vi "GetClampMAXResultValue.vi"(8 "error in (no error)":errorcluster, 9 "data":T1, 11 "Analysis_Clamp MAX_Parameter":T2) -> (0 "error out":errorcluster, 3 "ResultValues":string[](array[string]))   [LabVIEW 2019]
uses:
  Controls/Clamp MAX/Analysis_Clamp MAX_Parameter.ctl
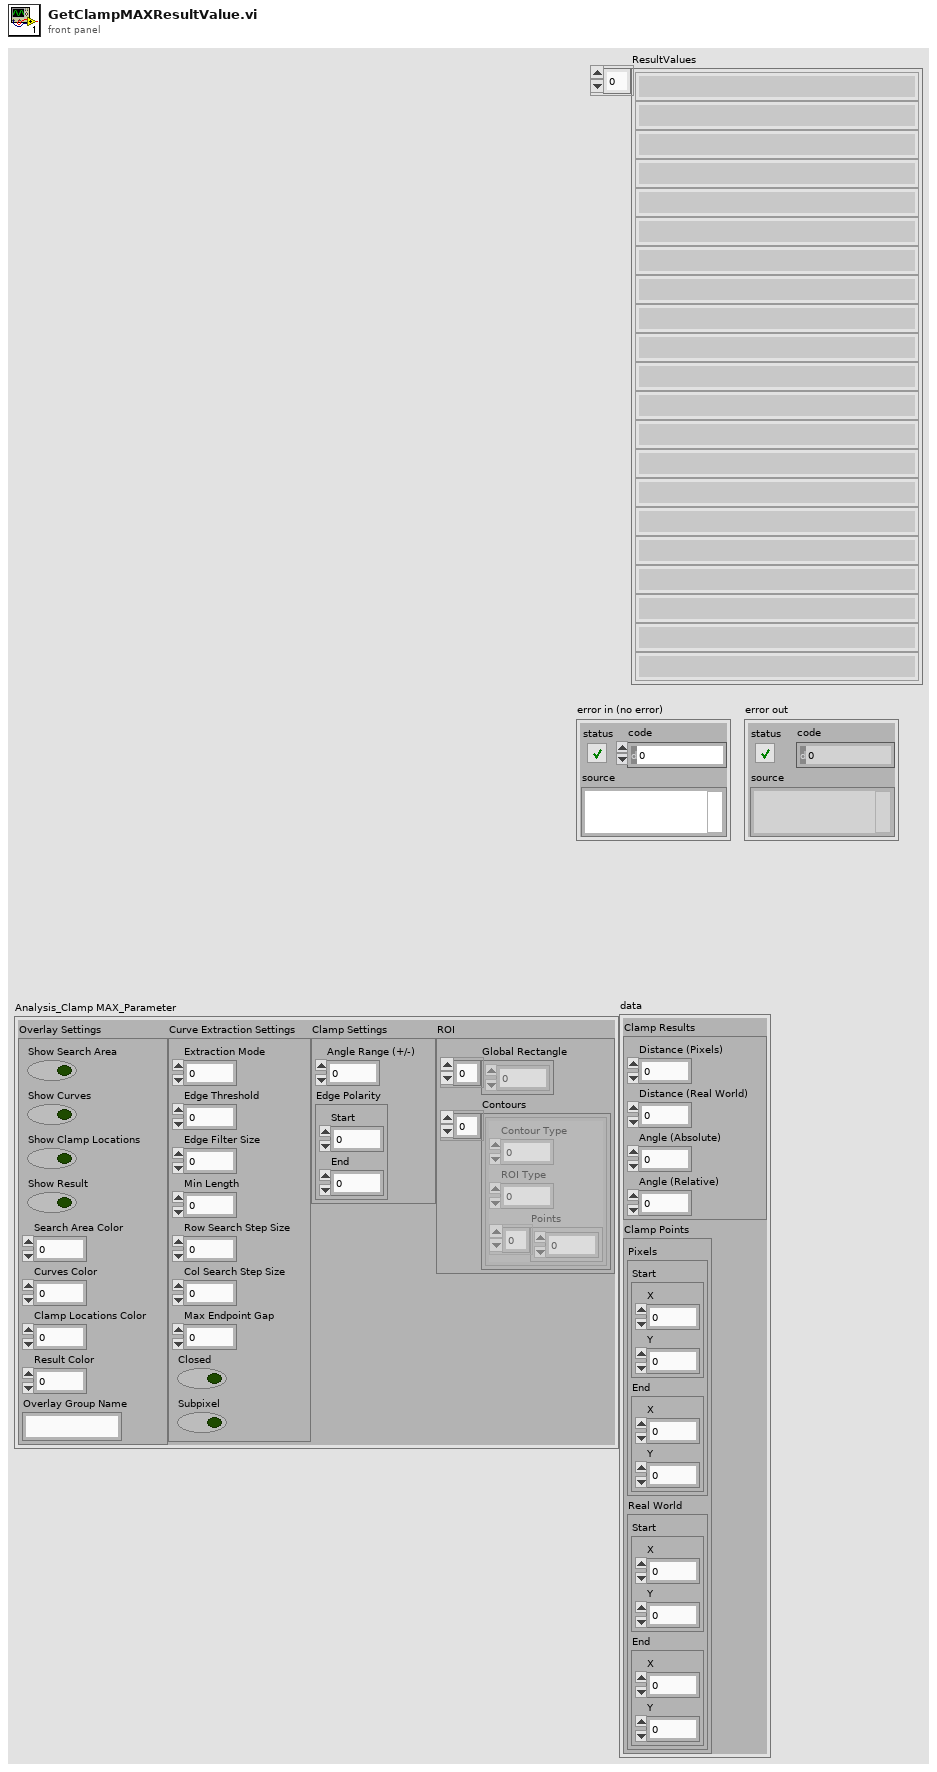
[diagram p1: front panel]
types:
  T1 = cluster{"Clamp Results":cluster{"Distance (Pixels)":dbl, "Distance (Real World)":dbl, "Angle (Absolute)":dbl, "Angle (Relative)":dbl}, "Clamp Points":cluster{"Pixels ":cluster{"Start":cluster{"X":dbl, "Y":dbl}, "End":cluster{"X":dbl, "Y":dbl}}, "Real World":cluster{"Start":cluster{"X":dbl, "Y":dbl}, "End":cluster{"X":dbl, "Y":dbl}}}}
  T2 = typedef "Analysis_Clamp MAX_Parameter.ctl" = cluster{"Overlay Settings":cluster{"Show Search Area":bool, "Show Curves":bool, "Show Clamp Locations":bool, "Show Result":bool, "Search Area Color":u32, "Curves Color":u32, "Clamp Locations Color":u32, "Result Color":u32, "Overlay Group Name":string}, "Curve Extraction Settings":cluster{"Extraction Mode":u32, "Edge Threshold":i32, "Edge Filter Size":u32, "Min Length":i32, "Row Search Step Size":i32, "Col Search Step Size":i32, "Max Endpoint Gap":i32, "Closed":bool, "Subpixel":bool}, "Clamp Settings":cluster{"Angle Range (+/-)":dbl, "Edge Polarity":cluster{"Start":u32, "End":u32}}, "ROI":cluster{"Global Rectangle":i32[], "Contours":cluster{"Contour Type":u32, "ROI Type":u32, "Points":i32[]}[]}}
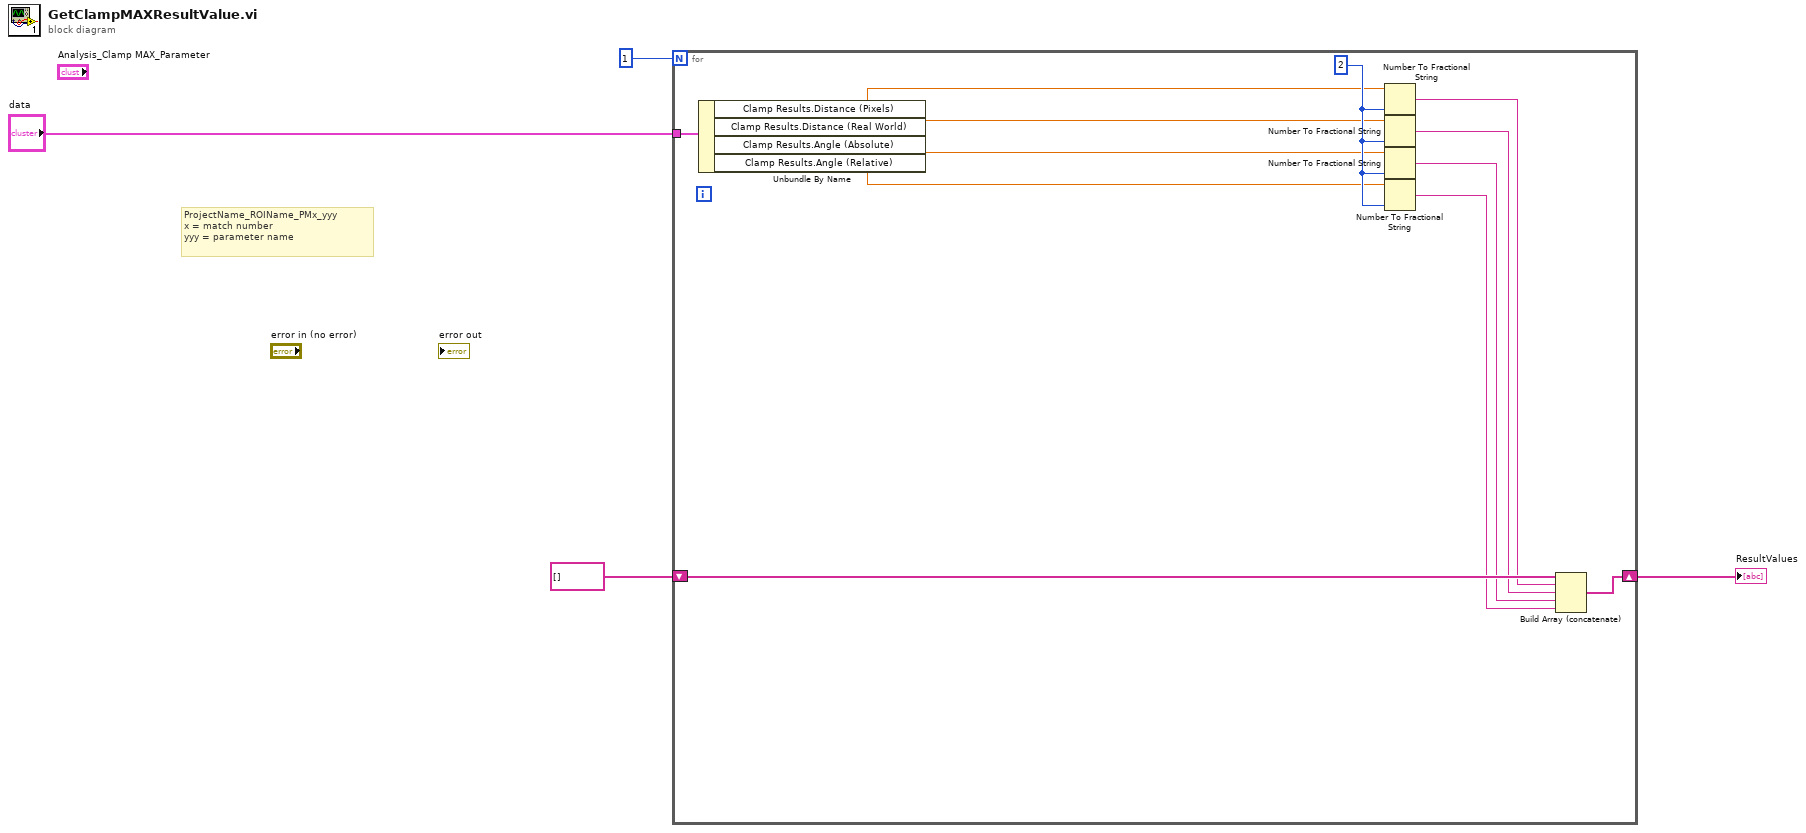
[diagram p0: block diagram]
diagram:
  # "ProjectName_ROIName_PMx_yyy\nx = match number\nyyy = parameter name"
  n1 = for {
    N: 1 ("Number of Matches Requested") -> [_]
    shift-right: [w10] -> w3
    shift-left: string[] [] -> [w15]
    tunnel: "data" -> [w16]
    w9 = 2
    n2 = Unbundle By Name(w16) -> ("Clamp Results.Distance (Pixels)"=w8:dbl, "Clamp Results.Distance (Real World)"=w7:dbl, "Clamp Results.Angle (Absolute)"=w6:dbl, "Clamp Results.Angle (Relative)"=w5:dbl)
    n3 = Number To Fractional String(number=w8, precision (6)=w9) -> (F-format string=w14:string)  [unwired: 2 in]
    n4 = Number To Fractional String(number=w7, precision (6)=w9) -> (F-format string=w13:string)  [unwired: 2 in]
    n5 = Number To Fractional String(number=w6, precision (6)=w9) -> (F-format string=w12:string)  [unwired: 2 in]
    n6 = Number To Fractional String(number=w5, precision (6)=w9) -> (F-format string=w11:string)  [unwired: 2 in]
    n7 = Build Array (concatenate)(w15, w14, w13, w12, w11) -> (w10:string[])
  }
  "ResultValues" <- w3
